vi "RS-485 single-address oneshot_noSerOpenClose.vi"(4 "Address":u8=1, 5 "Command":T1 items=["Retrieve all sensor data", "Retrieve CTA data only", "USB streaming enable", "USB streaming disable", "Retrieve EEPROM table", "Set address byte", "Get address byte", "Run self-test"], 7 "COM Port":refnum<visa-resource-name>) -> (0 "I/O error":errorcluster, 1 "Checksum ok":bool, 2 "Data":sgl[](array[numeric]), 3 "COM Port out":refnum<visa-resource-name>)   [LabVIEW 2017]
uses:
  ctls/Cmds.ctl
  ctls/USB Tx msg cluster.ctl
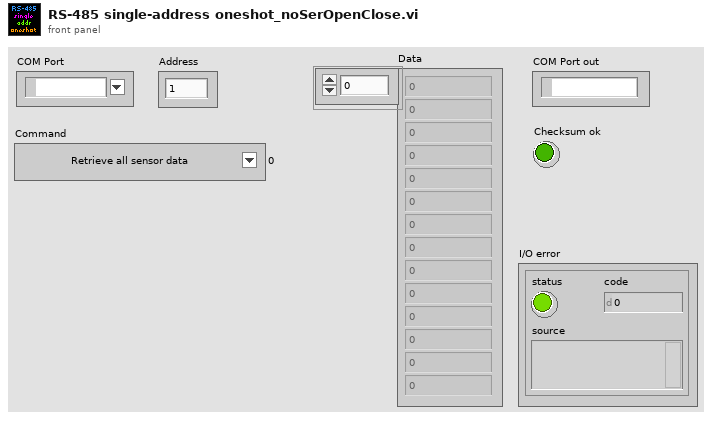
[diagram p1: front panel]
types:
  T1 = typedef "Cmds.ctl" = u8
  T2 = typedef "USB Tx msg cluster.ctl" = cluster{"addr":u8, "cmd":string, "data (float)":sgl}
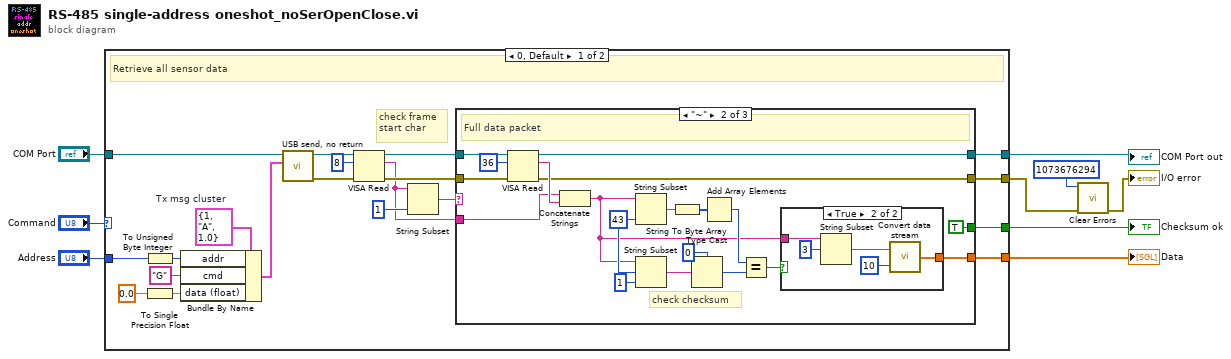
[diagram p0: block diagram]
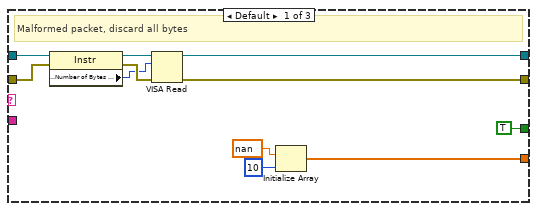
[diagram p2: hidden frame]
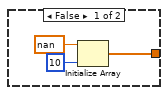
[diagram p3: hidden frame]
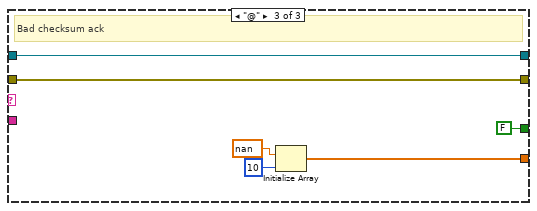
[diagram p4: hidden frame]
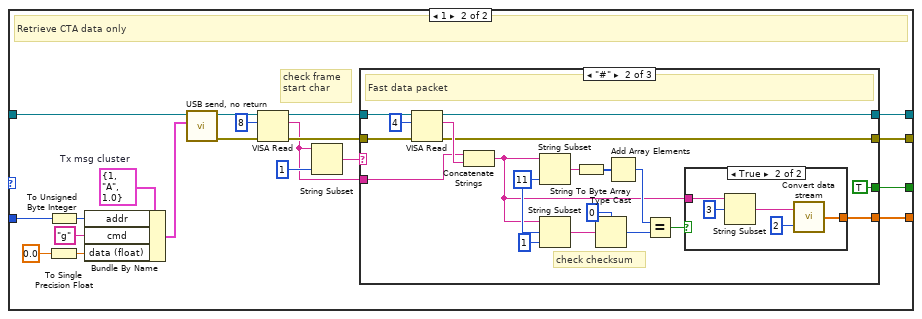
[diagram p5: hidden frame]
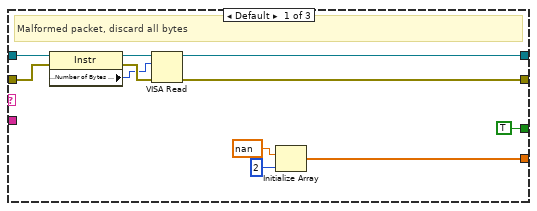
[diagram p6: hidden frame]
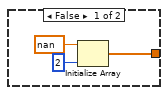
[diagram p7: hidden frame]
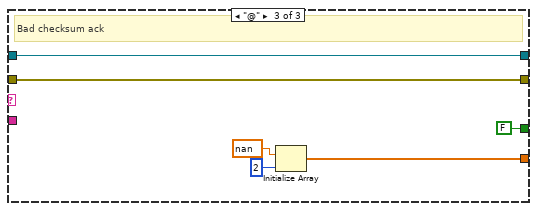
[diagram p8: hidden frame]
diagram:
  n1 = case shown="0, Default" "Command" {
    tunnel: "COM Port" -> [w29 w93]
    tunnel: [w25 w89] -> w2
    tunnel: [w28 w92] -> w1
    tunnel: [w27 w91] -> w7
    tunnel: "Address" -> [w26 w90]
    tunnel: [w24 w88] -> w4
    frame 0, Default {
      w21 = T2 {"addr"=1, "cmd"="A", "data (float)"=1.0}  # Tx msg cluster
      # "check frame start char"
      # "Retrieve all sensor data"
      n2 = To Unsigned Byte Integer(number=w26) -> (unsigned 8bit integer=w22:u8)
      n3 = To Single Precision Float(number=0.0) -> (single precision float=w23:sgl)
      n4 = Bundle By Name(cluster=w21, "addr"=w22, "cmd"="G", "data (float)"=w23) -> (w18:T2)
      n5 = call "USB send, no return.vi"("Tx msg cluster"=w18, "Port"=w29) -> ("Error out"=w13:errorcluster, "Port out"=w17:refnum<visa-resource-name>)  [unwired: 4 in]
      n6 = VISA Read(VISA resource name=w17, byte count=u32 8, error in (no error)=w13) -> (VISA resource name out=w15:refnum<visa-resource-name>, read buffer=w10:string, error out=w14:errorcluster)  [unwired: 1 out]
      n7 = String Subset(string=w10, length (rest)=1 ("length (rest)")) -> (substring=w11:string)  [unwired: 1 in]
      n8 = case shown="\"~\"" w11 {
        tunnel: [w38 w59 w72] -> w27
        tunnel: w15 -> [w32 w48 w71]
        tunnel: w14 -> [w31 w49 w70]
        tunnel: [w33 w44 w70] -> w25
        tunnel: [w34 w43 w71] -> w28
        tunnel: w10 -> [_ w42 _]
        tunnel: [TRUE TRUE FALSE] -> w24
        frame Default {
          # "Malformed packet, discard all bytes"
          n9 = property class="Instr"(reference=w32, error in=w31) -> (reference out=w37:refnum<visa-resource-name>, error out=w36:errorcluster, "Serial Settings:Number of Bytes at Serial Port"=w35:u32)
          n10 = VISA Read(VISA resource name=w37, byte count=w35, error in (no error)=w36) -> (VISA resource name out=w34:refnum<visa-resource-name>, error out=w33:errorcluster)  [unwired: 2 out]
          n11 = Initialize Array(sgl nan ("element"), 10 ("dimension size")) -> (w38:sgl[])
        }
        frame "~" {
          w56 = 43 ("length (rest)")
          # "check checksum"
          # "Full data packet"
          n12 = VISA Read(VISA resource name=w48, byte count=u32 36, error in (no error)=w49) -> (VISA resource name out=w43:refnum<visa-resource-name>, read buffer=w46:string, error out=w44:errorcluster)  [unwired: 1 out]
          n13 = Concatenate Strings(w42, w46) -> (w45:string)
          n14 = String Subset(string=w45, length (rest)=w56) -> (substring=w58:string)  [unwired: 1 in]
          n15 = String Subset(string=w45, offset (0)=w56, length (rest)=1 ("length (rest)")) -> (substring=w55:string)
          n16 = String To Byte Array(string=w58) -> (unsigned byte array=w57:u8[])
          n17 = Type Cast(type=u8 0 ("length (rest)"), x=w55) -> (*(type *) &x=w53:u8)
          n18 = Add Array Elements(numeric array=w57) -> (sum=w51:u8)
          n19 = Equal?(x=w51, y=w53) -> (x = y?=w52:bool)
          n20 = case shown="True" w52 {
            tunnel: [w60 w64] -> w59
            tunnel: w45 -> [_ w63]
            frame False {
              n21 = Initialize Array(sgl nan ("element"), 10 ("dimension size")) -> (w60:sgl[])
            }
            frame True {
              n22 = String Subset(string=w63, offset (0)=3) -> (substring=w66:string)  [unwired: 1 in]
              n23 = call "Convert data stream.vi"("n floats"=10, "Floats only (starting byte index 3)"=w66) -> ("Data"=w64:sgl[])
            }
          }
        }
        frame "@" {
          # "Bad checksum ack"
          n24 = Initialize Array(sgl nan ("element"), 10 ("dimension size")) -> (w72:sgl[])
        }
      }
    }
    frame 1 {
      w85 = T2 {"addr"=1, "cmd"="A", "data (float)"=1.0}  # Tx msg cluster
      # "check frame start char"
      # "Retrieve CTA data only"
      n25 = To Unsigned Byte Integer(number=w90) -> (unsigned 8bit integer=w86:u8)
      n26 = To Single Precision Float(number=0.0) -> (single precision float=w87:sgl)
      n27 = Bundle By Name(cluster=w85, "addr"=w86, "cmd"="g", "data (float)"=w87) -> (w82:T2)
      n28 = call "USB send, no return.vi"("Tx msg cluster"=w82, "Port"=w93) -> ("Error out"=w77:errorcluster, "Port out"=w81:refnum<visa-resource-name>)  [unwired: 4 in]
      n29 = VISA Read(VISA resource name=w81, byte count=u32 8, error in (no error)=w77) -> (VISA resource name out=w79:refnum<visa-resource-name>, read buffer=w74:string, error out=w78:errorcluster)  [unwired: 1 out]
      n30 = String Subset(string=w74, length (rest)=1 ("length (rest)")) -> (substring=w75:string)  [unwired: 1 in]
      n31 = case shown="\"#\"" w75 {
        tunnel: [w102 w123 w135] -> w91
        tunnel: w79 -> [w96 w112 w134]
        tunnel: w78 -> [w95 w113 w133]
        tunnel: [w97 w108 w133] -> w89
        tunnel: [w98 w107 w134] -> w92
        tunnel: w74 -> [_ w106 _]
        tunnel: [TRUE TRUE FALSE] -> w88
        frame Default {
          # "Malformed packet, discard all bytes"
          n32 = property class="Instr"(reference=w96, error in=w95) -> (reference out=w101:refnum<visa-resource-name>, error out=w100:errorcluster, "Serial Settings:Number of Bytes at Serial Port"=w99:u32)
          n33 = VISA Read(VISA resource name=w101, byte count=w99, error in (no error)=w100) -> (VISA resource name out=w98:refnum<visa-resource-name>, error out=w97:errorcluster)  [unwired: 2 out]
          n34 = Initialize Array(sgl nan ("element"), 2 ("dimension size")) -> (w102:sgl[])
        }
        frame "#" {
          w120 = 11 ("length (rest)")
          # "check checksum"
          # "Fast data packet"
          n35 = VISA Read(VISA resource name=w112, byte count=u32 4, error in (no error)=w113) -> (VISA resource name out=w107:refnum<visa-resource-name>, read buffer=w110:string, error out=w108:errorcluster)  [unwired: 1 out]
          n36 = Concatenate Strings(w106, w110) -> (w109:string)
          n37 = String Subset(string=w109, length (rest)=w120) -> (substring=w122:string)  [unwired: 1 in]
          n38 = String Subset(string=w109, offset (0)=w120, length (rest)=1 ("length (rest)")) -> (substring=w119:string)
          n39 = String To Byte Array(string=w122) -> (unsigned byte array=w121:u8[])
          n40 = Type Cast(type=u8 0 ("length (rest)"), x=w119) -> (*(type *) &x=w117:u8)
          n41 = Add Array Elements(numeric array=w121) -> (sum=w115:u8)
          n42 = Equal?(x=w115, y=w117) -> (x = y?=w116:bool)
          n43 = case shown="True" w116 {
            tunnel: [w124 w128] -> w123
            tunnel: w109 -> [_ w127]
            frame False {
              n44 = Initialize Array(sgl nan ("element"), 2 ("dimension size")) -> (w124:sgl[])
            }
            frame True {
              n45 = String Subset(string=w127, offset (0)=3) -> (substring=w130:string)  [unwired: 1 in]
              n46 = call "Convert data stream.vi"("n floats"=2, "Floats only (starting byte index 3)"=w130) -> ("Data"=w128:sgl[])
            }
          }
        }
        frame "@" {
          # "Bad checksum ack"
          n47 = Initialize Array(sgl nan ("element"), 2 ("dimension size")) -> (w135:sgl[])
        }
      }
    }
  }
  "Data" <- w7
  "Checksum ok" <- w4
  "COM Port out" <- w1
  n48 = call <vilib>:"Clear Errors.vi"("error in (no error)"=w2, "specific error code to clear (0: all)"=1073676294) -> ("error out"=→"I/O error":errorcluster)  [unwired: 4 in, 1 out]
